vi "Lot Begin.vi"(8 "error in":errorcluster, 10 "Test Result In":T2, 11 "CalCfg File In":T1) -> (0 "error out":errorcluster, 1 "Pass":bool, 2 "Test Result Out":T2, 3 "CalCfg File Out":T1, 4 "String":string)   [LabVIEW 2020, in "GUCalibration2.lvlib"]
uses:
  GUCalibration2.lvlib
  Controls/Test Result.ctl
  Controls/Site Data Element.ctl
  Controls/Site Raw Data Element.ctl
  Controls/CalibrationOrCheck.ctl
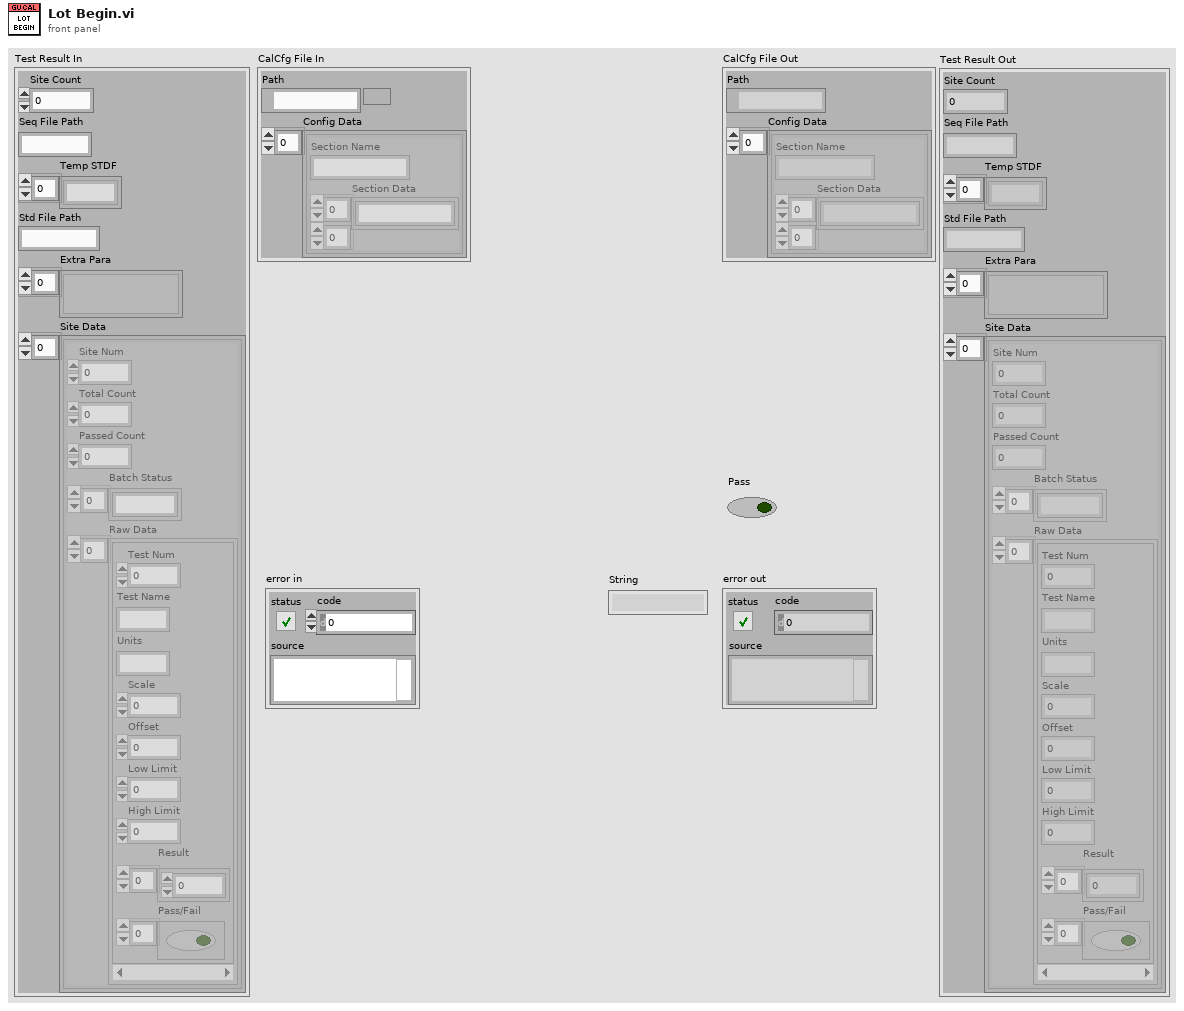
[diagram p1: front panel]
types:
  T1 = cluster{"Path":path, "Config Data":cluster{"Section Name":string, "Section Data":string[][]}[]}
  T2 = typedef "GUCalibration2.lvlib/Test Result.ctl" = cluster{"Site Count":i32, "Seq File Path":string, "Temp STDF":string[], "Std File Path":string, "Extra Para":variant[], "Site Data":T3[]}
  T3 = typedef "GUCalibration2.lvlib/Site Data Element.ctl" = cluster{"Site Num":i32, "Total Count":i32, "Passed Count":i32, "Batch Status":string[], "Raw Data":T4[]}
  T4 = typedef "GUCalibration2.lvlib/Site Raw Data Element.ctl" = cluster{"Test Num":u32, "Test Name":string, "Units":string, "Scale":i8, "Offset":dbl, "Low Limit":dbl, "High Limit":dbl, "Result":dbl[], "Pass/Fail":bool[]}
  T5 = typedef "GUCalibration2.lvlib/CalibrationOrCheck.ctl" = enum32{"Calibration", "Check"}
  T6 = cluster{"Section Name":string, "Section Data":string[][]}[]
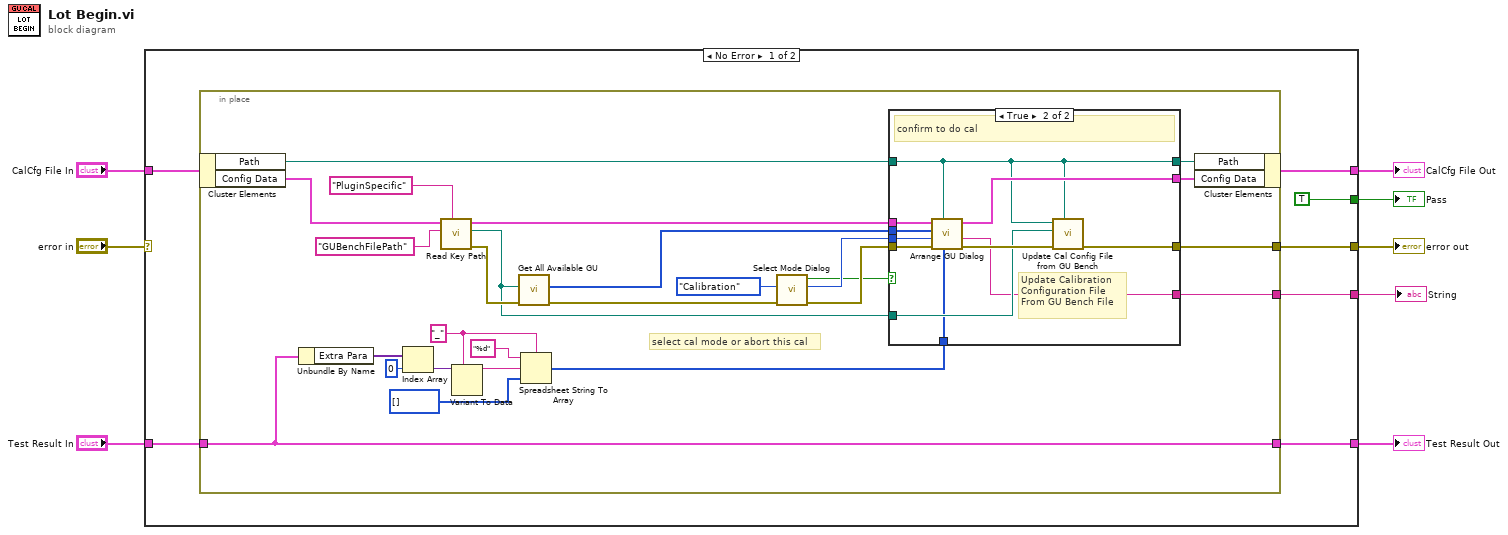
[diagram p0: block diagram]
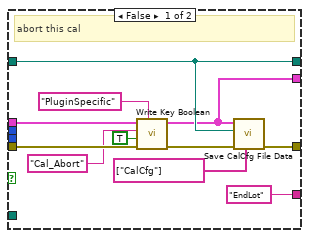
[diagram p2: hidden frame]
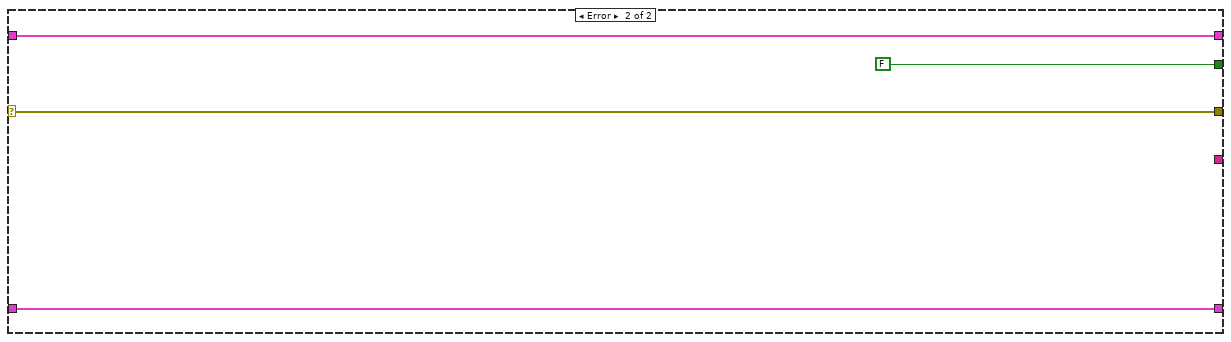
[diagram p3: hidden frame]
diagram:
  n1 = case shown="No Error" "error in" {
    selector: "error in" -> [_ w67]
    tunnel: [TRUE ("OK") FALSE ("OK")] -> w8
    tunnel: [w15 w67] -> w7
    tunnel: [w13 w66] -> w3
    tunnel: "CalCfg File In" -> [w14 w66]
    tunnel: "Test Result In" -> [w12 w64]
    tunnel: [w11 w64] -> w2
    tunnel: [w9 _] -> w1
    frame No Error {
      n2 = in-place {
        in-place-border: [w41] -> w15
        in-place-border: w12 -> [w40]
        in-place-border: [w40] -> w11
        in-place-border: [w26] -> w9
        w17 = "_" ("delimiter (Tab)")
        # "select cal mode or abort this cal"
        n3 = in-place-cluster #1(w14) -> ("Path"=w33:path, "Config Data"=w38:T6)
        n4 = Unbundle By Name(w40) -> ("Extra Para"=w18:variant[])
        n5 = Index Array(array=w18, index=0) -> (element=w22:variant)
        n6 = call "Read Key Path.vi"("Section Name"="PluginSpecific", "Key Names"="GUBenchFilePath" ("Section Name"), "Config Data"=w38) -> ("error out"=w36:errorcluster, "Key Value out"=w29:path, "Config Data dup"=w35:T6)  [unwired: 4 in, 2 out]
        n7 = Variant To Data(type=w17, Variant=w22) -> (data=w20:string)  [unwired: 1 in, 1 out]
        n8 = call "Get All Available GU.vi"("error in"=w36, "GU Bench File Path"=w29) -> ("error out"=w34:errorcluster, "GU Numbers Out"=w32:i32[])  [unwired: 8 in]
        n9 = Spreadsheet String To Array(delimiter (Tab)=w17, format string="%d", spreadsheet string=w20, array type (2D Dbl)=i32[] []) -> (array=w27:i32[])
        n10 = call "Select Mode Dialog.vi"("error in"=w34, "Comp/Check in"=CalibrationOrCheck."Calibration" ("Comp/Check")) -> ("error out"=w31:errorcluster, "Comp/Check out"=w30:T5, "OK?"=w24:bool)  [unwired: 7 in]
        n11 = case shown="True" w24 {
          tunnel: [w51 w63] -> w41
          tunnel: w35 -> [w45 w62]
          tunnel: w33 -> [w50 w53]
          tunnel: w32 -> [_ w61]
          tunnel: w31 -> [w48 w60]
          tunnel: w30 -> [_ w59]
          tunnel: w29 -> [_ w57]
          tunnel: [w44 w56] -> w28
          tunnel: w27 -> [_ w55]
          tunnel: ["EndLot" ("Msg") w54] -> w26
          tunnel: [w50 w53] -> w25
          frame False {
            # "abort this cal"
            n12 = call "Write Key Boolean.vi"("Section Name"="PluginSpecific", "error in (no error)"=w48, "Key Value"=TRUE, "Key Name"="Cal_Abort" ("Section Name"), "Config Data"=w45) -> ("error out"=w47:errorcluster, "Config Data dup"=w44:T6)  [unwired: 5 in]
            n13 = call "Save CalCfg File Data.vi"("Matric Section"=string[] ["CalCfg"], "error in"=w47, "File Path"=w50, "Config Data"=w44) -> ("error out"=w51:errorcluster)  [unwired: 7 in]
          }
          frame True {
            # "Update Calibration\nConfiguration File\nFrom GU Bench File"
            # "confirm to do cal"
            n14 = call "Arrange GU Dialog.vi"("Enabled Site"=w55, "CAL Config File Path"=w53, "error in"=w60, "Cur Cal Type"=w59, "All Available GU"=w61, "Config File Data"=w62) -> ("error out"=w58:errorcluster, "Msg"=w54:string, "Config File.Data"=w56:T6)  [unwired: 3 in]
            n15 = call "Update Cal Config File from GU Bench.vi"("Output File Path"=w53, "error in"=w58, "GU Bench File Path"=w57, "Calibration Config File Path"=w53) -> ("error out"=w63:errorcluster)  [unwired: 7 in]
          }
        }
        n16 = in-place-cluster #1("Path"=w25, "Config Data"=w28) -> (w13:T1)
      }
    }
    frame Error {
    }
  }
  "error out" <- w7
  "Pass" <- w8
  "Test Result Out" <- w2
  "CalCfg File Out" <- w3
  "String" <- w1
